vi "loginInfo(SubVI).vi"(0 "connection reference 2":T1) -> (1 "connection reference 4":T1, 2 "GetUserName 3":string[](array[string]), 3 "GetAdminNo 3":string[](array[string]), 4 "GetPassword 3":string[](array[string]))   [LabVIEW 2013]
uses:
  <vilib>/addons/database/Connection.llb/Conn ObjectReference.ctl
  <vilib>/addons/database/_DB Variant To Data/Database Variant To Data.xnode
  <vilib>/addons/database/NI_Database_API.lvlib
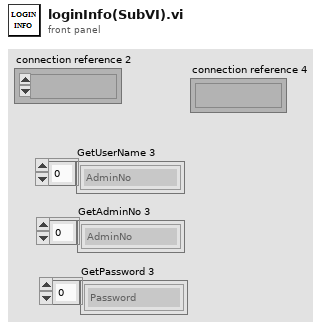
[diagram p1: front panel]
types:
  T1 = typedef "NI_Database_API.lvlib/Conn ObjectReference.ctl" = refnum<k1>
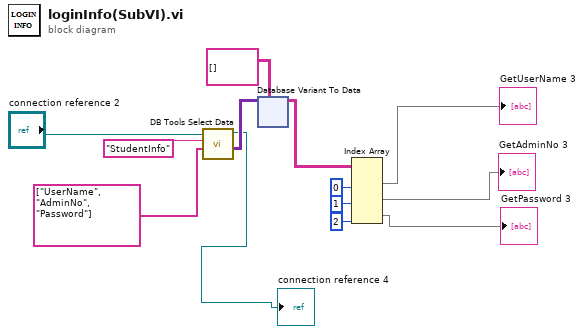
[diagram p0: block diagram]
diagram:
  n1 = call <vilib>:"DB Tools Select Data.vi"("columns"=string[] ["UserName", "AdminNo", "Password"], "table"="StudentInfo", "connection reference"="connection reference 2") -> ("data"=w13:variant[][], "connection reference out"=→"connection reference 4":T1)  [unwired: 3 in, 1 out]
  n2 = xnode "Database Variant To Data"("database variant"=w13, "type"=string[][] [] ("data")) -> ("data"=w9:string[][])  [unwired: 1 in, 1 out]
  n3 = Index Array(array=w9, index (col) #1=0 ("disabled index (col)"), index (col) #2=1 ("index (col)"), index (col) #3=2 ("index (col)")) -> (element #1=→"GetUserName 3":string[], element #2=→"GetAdminNo 3":string[], element #3=→"GetPassword 3":string[])  [unwired: 3 in]
